vi "Trigger.vi"(8 "error in (no error)":errorcluster, 11 "Red Pitaya Digitizer in":refnum<class "Red Pitaya Digitizer.lvclass">) -> (0 "error out":errorcluster, 3 "Red Pitaya Digitizer out":refnum<class "Red Pitaya Digitizer.lvclass">)   [LabVIEW 2016, in "Red Pitaya Digitizer.lvclass"]
uses:
  Red Pitaya Digitizer.lvclass
  Red Pitaya Digitizer.lvclass/Red Pitaya Digitizer.ctl
  Read RP Instrument.vi
  Write RP Instrument.vi
  RP Core/RP Instrument/RP Instrument.lvclass
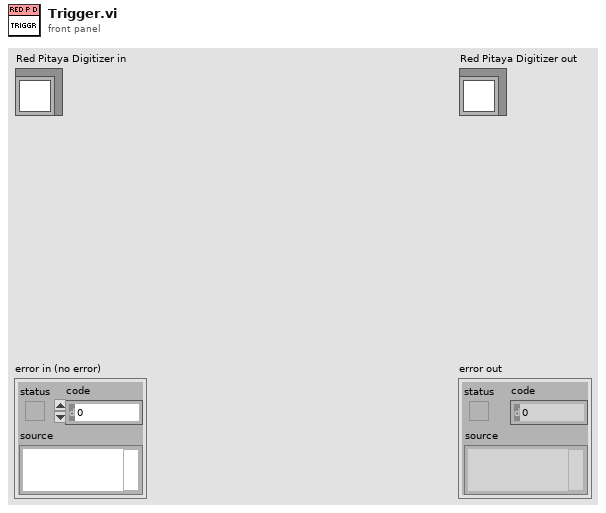
[diagram p1: front panel]
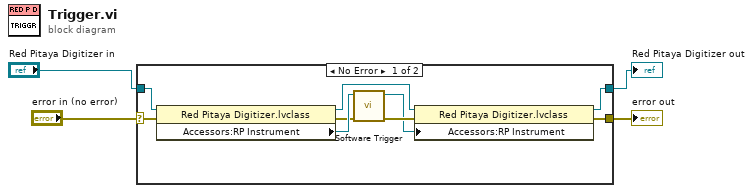
[diagram p0: block diagram]
diagram:
  n1 = case shown="No Error" "error in (no error)" {
    selector: "error in (no error)" -> [w10 w15]
    tunnel: "Red Pitaya Digitizer in" -> [w13 w14]
    tunnel: [w6 w14] -> w1
    tunnel: [w5 w15] -> w3
    frame No Error {
      n2 = property class="Red Pitaya Digitizer.lvclass"(reference=w13, error in=w10) -> (reference out=w9:refnum<class "Red Pitaya Digitizer.lvclass">, error out=w11:errorcluster, "Accessors:RP Instrument"=w12:refnum<class "RP Instrument.lvclass">)
      n3 = call-dynamic "Software Trigger.vi"("error in (no error)"=w11, "RP Instrument in"=w12) -> ("error out"=w8:errorcluster, "RP Instrument out"=w7:refnum<class "RP Instrument.lvclass">)  [unwired: 8 in]
      n4 = property class="Red Pitaya Digitizer.lvclass"(reference=w9, error in=w8, "Accessors:RP Instrument"=w7) -> (reference out=w6:refnum<class "Red Pitaya Digitizer.lvclass">, error out=w5:errorcluster)
    }
    frame Error {
    }
  }
  "error out" <- w3
  "Red Pitaya Digitizer out" <- w1
